vi "sense iv(k).vi"() -> ()   [LabVIEW 2017]
doc: "This example shows how to create, run a script and query the script output data."
uses:
  <instrlib>/Keithley 2600 Series/Keithley 2600 Series.lvlib
panel:
  out "Power":dbl
  out "Time Stamp":string[](array[string])
  out "Current(A)":dbl
  out "Voltage(V)":dbl
  in  "SweepSetting":T1={"CurrentLimit(A)"=0.1, "Start Voltage(V)"=0.0} {"Start Voltage(V)" min=-200.0 max=200.0; "CurrentLimit(A)" min=1e-09 max=1.5}
  in  "USB COM Port":refnum<visa-resource-name>="COM5"
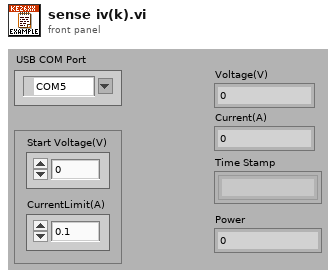
[diagram p1: front panel]
types:
  T1 = cluster{"CurrentLimit(A)":dbl, "Start Voltage(V)":dbl}
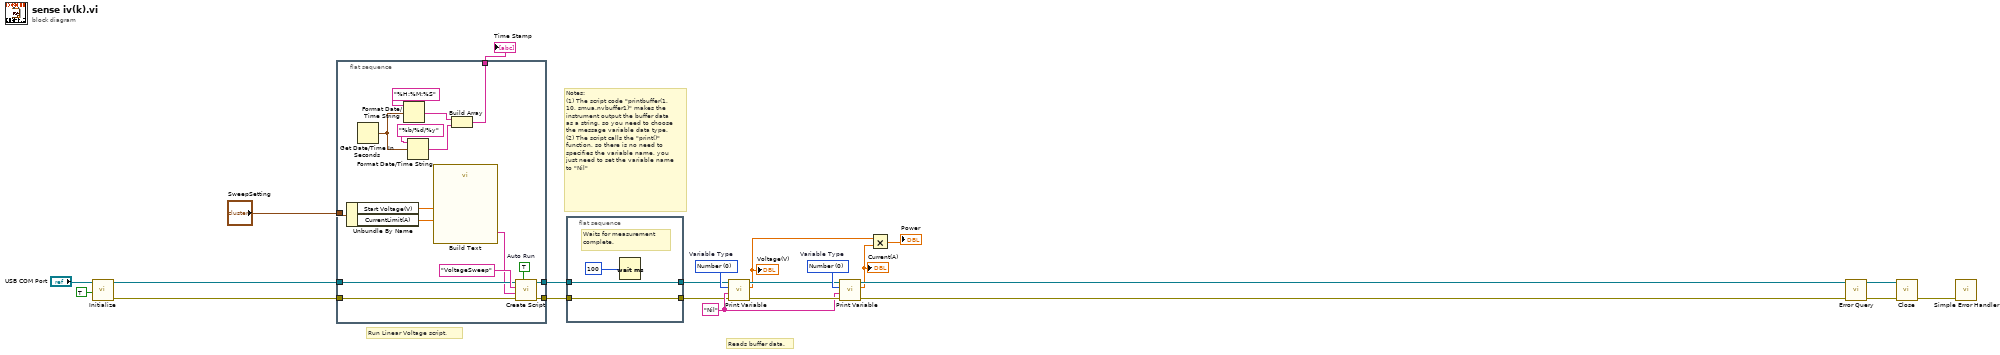
[diagram p0: block diagram]
diagram:
  w7 = "Nil"
  w12 = 0 items=["Number", "Message"]  # Variable Type
  w13 = 0 items=["Number", "Message"]  # Variable Type
  # "Reads buffer data."
  # "Notes: \n(1) The script code \"printbuffer(1, 10, smua.nvbuffer1)\" makes the instrument output the buffer data as a string, so you need to choose the message variable data type.\n(2) The script calls the \"print()\" function, so there is no need to specifies the variable name, you just need to set the variable name to \"Nil\""
  # "Run Linear Voltage script."
  n1 = call <instrlib>:"Initialize.vi"("Reset (True)"=TRUE, "VISA resource name"="USB COM Port") -> ("error out"=w16:errorcluster, "VISA resource name out"=w17:refnum<visa-resource-name>)  [unwired: 8 in]
  n2 = flat-sequence {
    tunnel: [w37] -> w22
    tunnel: [w36] -> w21
    tunnel: w17 -> [w35]
    tunnel: w16 -> [w34]
    tunnel: "SweepSetting" -> [w32]
    tunnel: [w26] -> w2
    frame #0 {
      w38 = TRUE  # Auto Run
      n3 = Unbundle By Name(w32) -> ("Start Voltage(V)"=w24:dbl, "CurrentLimit(A)"=w25:dbl)
      n4 = Get Date/Time In Seconds() -> (seconds since 1Jan1904=w27:timestamp)
      n5 = Format Date/Time String(time format string (%c)="%H:%M:%S", seconds (now)=w27) -> (date/time string=w30:string)  [unwired: 1 out]
      n6 = Format Date/Time String(time format string (%c)="%b/%d/%y", seconds (now)=w27) -> (date/time string=w28:string)  [unwired: 1 out]
      n7 = call "Build Text"("limitI"=w25, "volt"=w24) -> ("Result"=w33:string)  [unwired: 12 in, 1 out]
      n8 = Build Array(w30, w28) -> (w26:string[])
      n9 = call <instrlib>:"Create Script.vi"("Auto Run (F: Disable)"=w38, "error in (no error)"=w34, "Source Code"=w33, "Script Variable"="VoltageSweep" ("Script Variable (myScript)"), "VISA resource name"=w35) -> ("error out"=w36:errorcluster, "VISA resource name out"=w37:refnum<visa-resource-name>)  [unwired: 5 in]
    }
  }
  n10 = flat-sequence {
    tunnel: w22 -> [w40]
    tunnel: w21 -> [w41]
    tunnel: [w41] -> w5
    tunnel: [w40] -> w6
    frame #0 {
      # "Waits for measurement complete."
      n11 = Wait (ms)(milliseconds to wait=100 ("Temp Delay")) -> ()  [unwired: 1 out]
    }
  }
  n12 = call <instrlib>:"Print Variable.vi"("error in (no error)"=w5, "Variable Name"=w7, "Variable Type (0: Number)"=w13, "VISA resource name"=w6) -> ("error out"=w10:errorcluster, "Number"=w3:dbl, "VISA resource name out"=w11:refnum<visa-resource-name>)  [unwired: 4 in, 1 out]
  "Voltage(V)" <- w3
  n13 = call <instrlib>:"Print Variable.vi"("error in (no error)"=w10, "Variable Name"=w7, "Variable Type (0: Number)"=w12, "VISA resource name"=w11) -> ("error out"=w8:errorcluster, "Number"=w4:dbl, "VISA resource name out"=w9:refnum<visa-resource-name>)  [unwired: 4 in, 1 out]
  "Current(A)" <- w4
  n14 = Multiply(x=w3, y=w4) -> (x*y=→"Power":dbl)
  n15 = call <instrlib>:"Error Query.vi"("error in (no error)"=w8, "VISA resource name"=w9) -> ("error out"=w19:errorcluster, "VISA resource name out"=w20:refnum<visa-resource-name>)  [unwired: 6 in, 2 out]
  n16 = call <instrlib>:"Close.vi"("error in (no error)"=w19, "VISA resource name"=w20) -> ("error out"=w23:errorcluster)  [unwired: 9 in]
  n17 = call <vilib>:"Simple Error Handler.vi"("error in (no error)"=w23) -> ()  [unwired: 4 in, 5 out]
  "Time Stamp" <- w2
